vi "Configure Modulation (Phase).vi"(0 "VISA resource name":refnum<visa-resource-name>, 1 "Enable Phase Modulation (T: Enable)":bool=TRUE, 5 "Channel (0: Channel 1)":T1 items=["Channel 1", "Channel 2"], 7 "PM Source (0: Internal)":u16(ring) items=["Internal", "External"], 9 "Modulation Waveform (0: Sine)":u16(ring) items=["Sine", "Square", "Triangle", "Ramp", "Down Ramp", "Noise"], 11 "error in (no error)":errorcluster, 12 "Modulation Frequency (100.00 Hz)":dbl[unit]=100.0 format="%#_6f", 13 "Peak Deviation (90 deg)":dbl=90.0 min=-180.0 max=180.0 format="%#.4f") -> (4 "VISA resource name out":refnum<visa-resource-name>, 15 "error out":errorcluster)   [LabVIEW 2009, in "Tektronix AFG 3000 Series.lvlib"]
doc: "Configures and enables phase modulation (PM). In PM, the phase of the carrier is varied by the peak deviation and the modulating waveform. \n\n<B>Note:</B>\n\nDefault measure for peak deviation is in degrees only. To change deviation unit to radians replace the DEG with RAD in the peak deviation command.\n\n***NOTE: this likely doesn't correctly go back to internal if you set it to external. See \"Configure Modulation (Amplitude).vi\" for how to fix it, if needed."
uses:
  Tektronix AFG 3000 Series.lvlib
  controls.llb/Channel.ctl
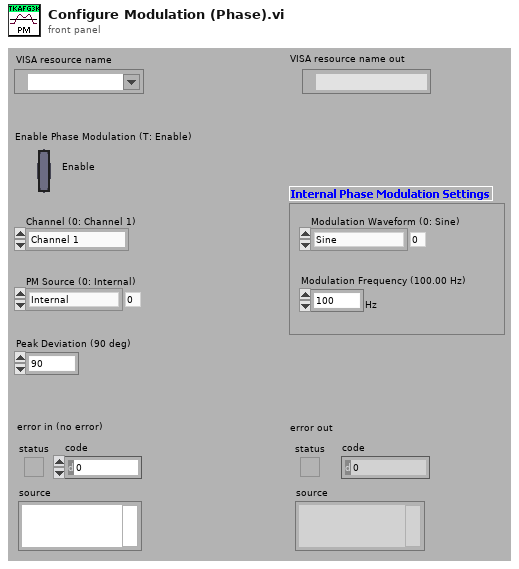
[diagram p1: front panel]
types:
  T1 = typedef "Channel.ctl" = u16
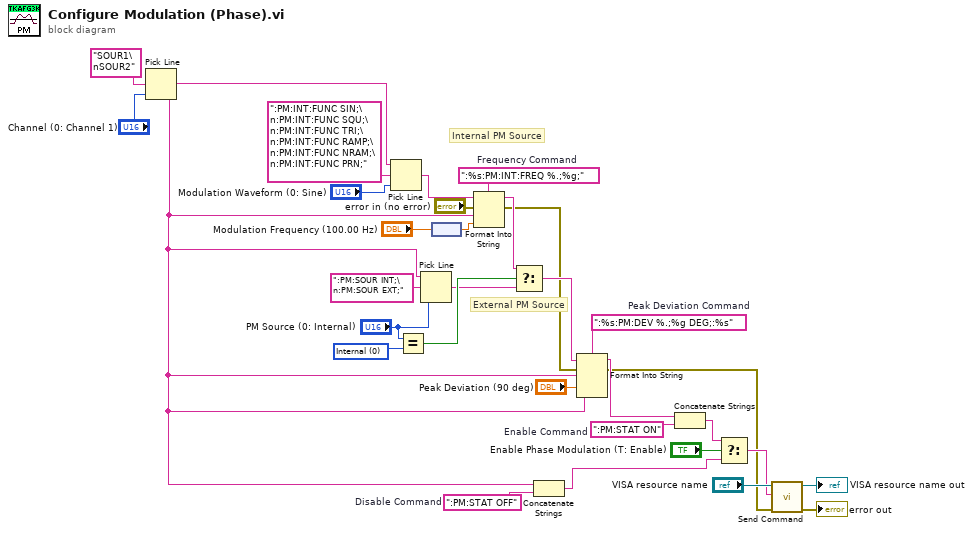
[diagram p0: block diagram]
diagram:
  w17 = ":%s:PM:INT:FREQ %.;%g;"  # Frequency Command
  w26 = ":PM:STAT ON"  # Enable Command
  w28 = ":%s:PM:DEV %.;%g DEG;:%s"  # Peak Deviation Command
  w30 = u16 0 items=["Internal", "External"] ("Source (0: Internal)")
  w22 = ":PM:STAT OFF"  # Disable Command
  # "External PM Source"
  # "Internal PM Source"
  n1 = Pick Line(multi-line string="SOUR1\nSOUR2" ("string (\"\")"), line index="Channel (0: Channel 1)") -> (output string=w10:string)  [unwired: 1 out]
  n2 = Pick Line(string ("")=w10, multi-line string=":PM:INT:FUNC SIN;\n:PM:INT:FUNC SQU;\n:PM:INT:FUNC TRI;\n:PM:INT:FUNC RAMP;\n:PM:INT:FUNC NRAM;\n:PM:INT:FUNC PRN;", line index="Modulation Waveform (0: Sine)") -> (output string=w18:string)
  n3 = Equal?(x="PM Source (0: Internal)", y=w30) -> (x = y?=w16:bool)
  n4 = Pick Line(string ("")=w10, multi-line string=":PM:SOUR INT;\n:PM:SOUR EXT;" ("Source Command"), line index="PM Source (0: Internal)") -> (output string=w15:string)
  n5 = node("Modulation Frequency (100.00 Hz)") -> (w6:dbl)
  n6 = Format Into String(format string=w17, initial string=w18, error in="error in (no error)", w10, w6) -> (resulting string=w14:string, error out=w8:errorcluster)
  n7 = Select(t=w14, s=w16, f=w15) -> (s? t:f=w13:string)
  n8 = Concatenate Strings(w10, w22) -> (w20:string)
  n9 = Format Into String(format string=w28, initial string=w13, error in=w8, w10, "Peak Deviation (90 deg)", w10) -> (resulting string=w27:string, error out=w2:errorcluster)
  n10 = Concatenate Strings(w27, w26) -> (w12:string)
  n11 = Select(t=w12, s="Enable Phase Modulation (T: Enable)", f=w20) -> (s? t:f=w3:string)
  n12 = call "Send Command.vi"("error in (no error)"=w2, "write buffer"=w3, "VISA resource name"="VISA resource name") -> ("error out"=→"error out":errorcluster, "VISA resource name out"=→"VISA resource name out":refnum<visa-resource-name>)  [unwired: 7 out]
